vi "StatusReq20.vi"(1 "aDATA in":u8[](array[numeric])) -> ()   [LabVIEW 2017]
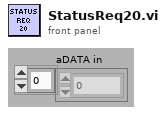
[diagram p1: front panel]
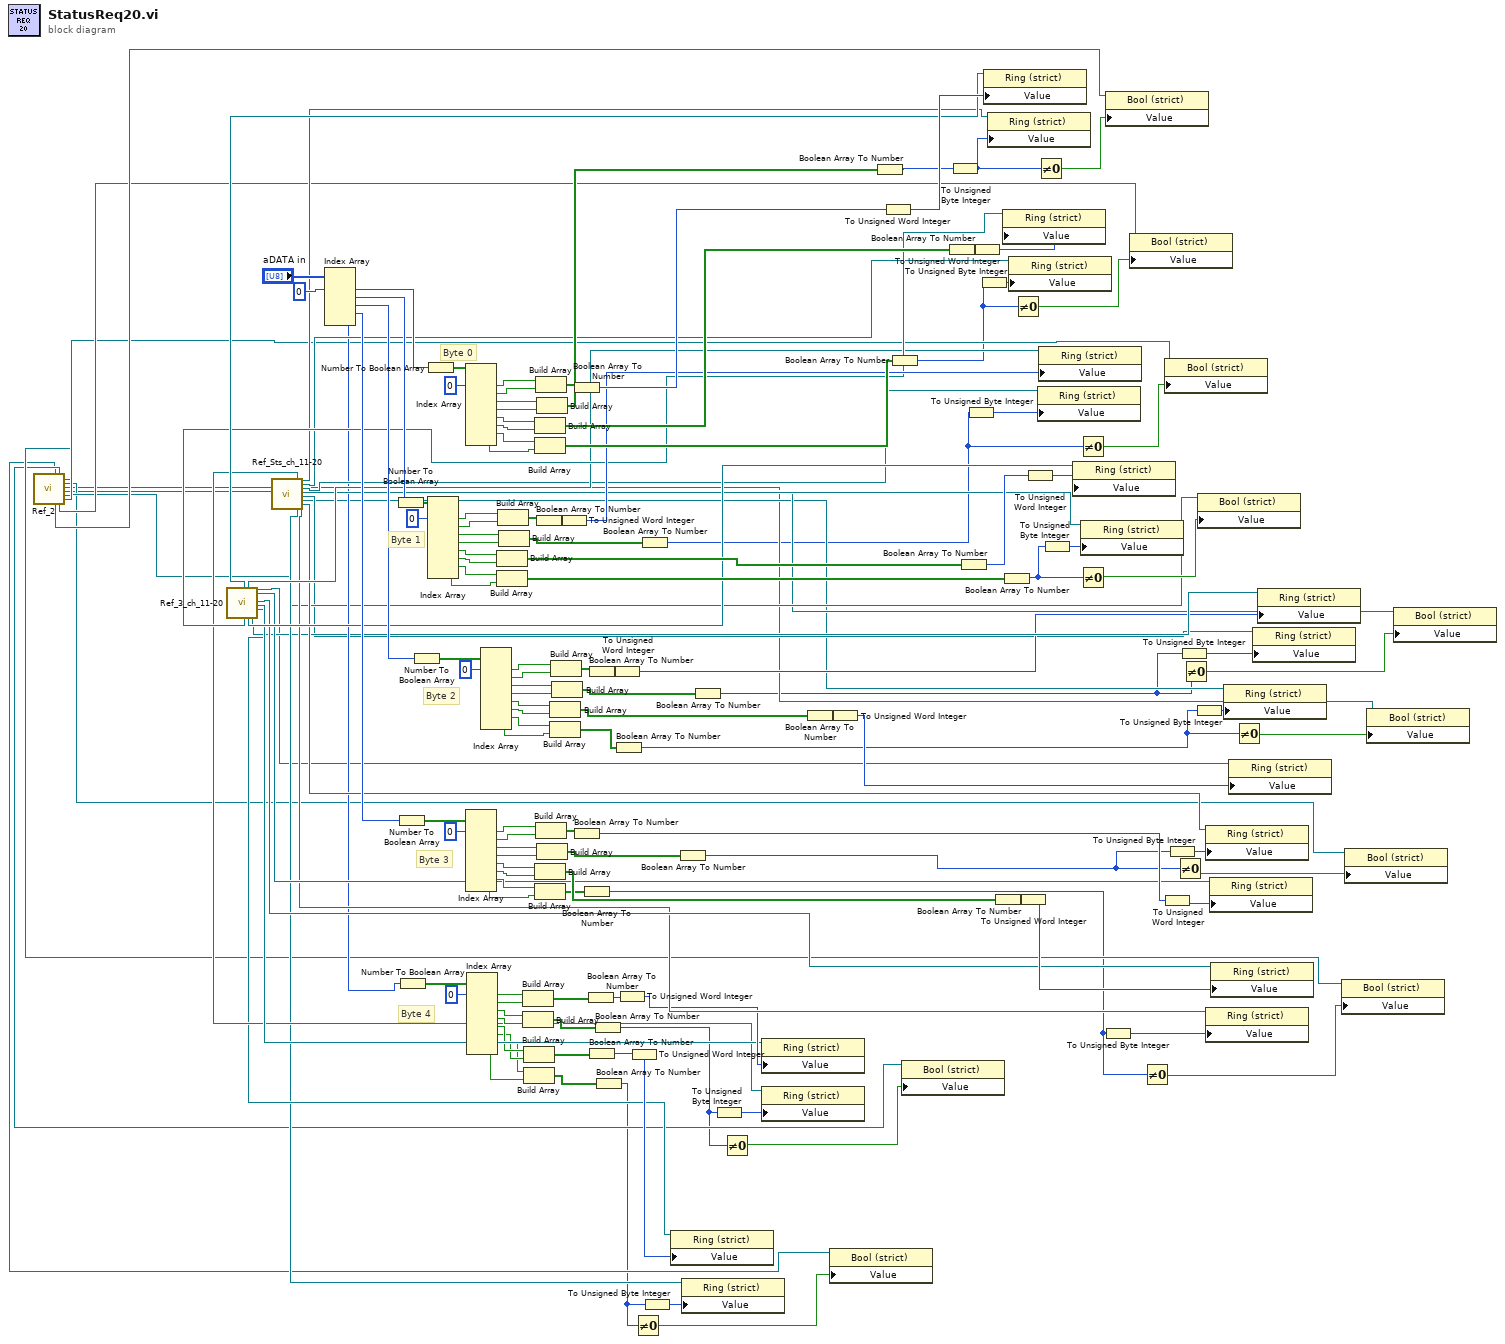
[diagram p0: block diagram]
diagram:
  # "Byte 4"
  # "Byte 3"
  # "Byte 2"
  # "Byte 1"
  # "Byte 0"
  n1 = call "Ref_2.vi"() -> ("Control  Ch 10 out"=w32:refnum<vi>, "Control  Ch 1 out"=w39:refnum<vi>, "Control  Ch 9 out"=w33:refnum<vi>, "Control  Ch 2 out"=w38:refnum<vi>, "Control  Ch 8 out"=w34:refnum<vi>, "Control  Ch 7 out"=w35:refnum<vi>, "Control  Ch 6 out"=w22:refnum<vi>, "Control  Ch 5 out"=w27:refnum<vi>, "Control  Ch 4 out"=w36:refnum<vi>, "Control  Ch 3 out"=w37:refnum<vi>)  [unwired: 17 in, 1 out]
  n2 = call "Ref_3_ch_11-20.vi"() -> ("Trip  Ch 11 out"=w81:refnum<vi>, "Trip  Ch 12 out"=w80:refnum<vi>, "Trip  Ch 13 out"=w79:refnum<vi>, "Trip  Ch 14 out"=w78:refnum<vi>, "Trip  Ch 15 out"=w31:refnum<vi>, "Trip  Ch 16 out"=w23:refnum<vi>, "Trip  Ch 17 out"=w77:refnum<vi>, "Trip  Ch 18 out"=w76:refnum<vi>, "Trip  Ch 19 out"=w58:refnum<vi>, "Trip  Ch 20 out"=w48:refnum<vi>)  [unwired: 18 in]
  n3 = call "Ref_Sts_ch_11-20.vi"() -> ("Status Ch 19 out"=w57:refnum<vi>, "Status Ch 20 out"=w47:refnum<vi>, "Status Ch 11 out"=w75:refnum<vi>, "Status Ch 12 out"=w74:refnum<vi>, "Status Ch 13 out"=w73:refnum<vi>, "Status Ch 14 out"=w72:refnum<vi>, "Status Ch 15 out"=w28:refnum<vi>, "Status Ch 16 out"=w24:refnum<vi>, "Status Ch 17 out"=w71:refnum<vi>, "Status Ch 18 out"=w70:refnum<vi>)  [unwired: 18 in]
  n4 = Index Array(array="aDATA in", index #1=0 ("index")) -> (element #1=w155:u8, element #2=w117:u8, element #3=w116:u8, element #4=w115:u8, element #5=w67:u8)  [unwired: 4 in]
  n5 = Number To Boolean Array(number=w117) -> (Boolean array=w135:bool[])
  n6 = Number To Boolean Array(number=w115) -> (Boolean array=w118:bool[])
  n7 = Number To Boolean Array(number=w67) -> (Boolean array=w69:bool[])
  n8 = Number To Boolean Array(number=w116) -> (Boolean array=w134:bool[])
  n9 = Number To Boolean Array(number=w155) -> (Boolean array=w154:bool[])
  n10 = Index Array(array=w135, index #1=0 ("index")) -> (element #1=w106:bool, element #2=w105:bool, element #3=w104:bool, element #4=w103:bool, element #5=w102:bool, element #6=w101:bool, element #7=w100:bool, element #8=w99:bool)  [unwired: 7 in]
  n11 = Index Array(array=w154, index #1=0 ("index")) -> (element #1=w114:bool, element #2=w113:bool, element #3=w112:bool, element #4=w111:bool, element #5=w110:bool, element #6=w109:bool, element #7=w108:bool, element #8=w107:bool)  [unwired: 7 in]
  n12 = Index Array(array=w118, index #1=0 ("index")) -> (element #1=w90:bool, element #2=w89:bool, element #3=w88:bool, element #4=w87:bool, element #5=w86:bool, element #6=w85:bool, element #7=w84:bool, element #8=w83:bool)  [unwired: 7 in]
  n13 = Index Array(array=w69, index #1=0 ("index")) -> (element #1=w65:bool, element #2=w66:bool, element #3=w64:bool, element #4=w63:bool, element #5=w52:bool, element #6=w51:bool, element #7=w50:bool, element #8=w49:bool)  [unwired: 7 in]
  n14 = Index Array(array=w134, index #1=0 ("index")) -> (element #1=w98:bool, element #2=w97:bool, element #3=w96:bool, element #4=w95:bool, element #5=w94:bool, element #6=w93:bool, element #7=w92:bool, element #8=w91:bool)  [unwired: 7 in]
  n15 = Build Array(w102, w101) -> (w143:bool[])
  n16 = Build Array(w100, w99) -> (w142:bool[])
  n17 = Build Array(w106, w105) -> (w137:bool[])
  n18 = Build Array(w104, w103) -> (w144:bool[])
  n19 = Build Array(w65, w66) -> (w61:bool[])
  n20 = Build Array(w64, w63) -> (w60:bool[])
  n21 = Build Array(w52, w51) -> (w54:bool[])
  n22 = Build Array(w50, w49) -> (w55:bool[])
  n23 = Boolean Array To Number(Boolean array=w137) -> (number=w138:u32)
  n24 = Build Array(w110, w109) -> (w146:bool[])
  n25 = Build Array(w108, w107) -> (w147:bool[])
  n26 = Build Array(w86, w85) -> (w125:bool[])
  n27 = Build Array(w84, w83) -> (w82:bool[])
  n28 = Build Array(w114, w113) -> (w152:bool[])
  n29 = Build Array(w90, w89) -> (w120:bool[])
  n30 = Build Array(w112, w111) -> (w145:bool[])
  n31 = Build Array(w88, w87) -> (w126:bool[])
  n32 = Build Array(w94, w93) -> (w128:bool[])
  n33 = Build Array(w92, w91) -> (w129:bool[])
  n34 = Build Array(w98, w97) -> (w132:bool[])
  n35 = Build Array(w96, w95) -> (w127:bool[])
  n36 = To Unsigned Word Integer(number=w138) -> (unsigned 16bit integer=w139:u16)
  n37 = Boolean Array To Number(Boolean array=w152) -> (number=w151:u32)
  n38 = Boolean Array To Number(Boolean array=w120) -> (number=w121:u32)
  n39 = Boolean Array To Number(Boolean array=w82) -> (number=w6:u32)
  n40 = Boolean Array To Number(Boolean array=w61) -> (number=w62:u32)
  n41 = Boolean Array To Number(Boolean array=w132) -> (number=w131:u32)
  n42 = Boolean Array To Number(Boolean array=w54) -> (number=w53:u32)
  n43 = Boolean Array To Number(Boolean array=w60) -> (number=w4:u32)
  n44 = Boolean Array To Number(Boolean array=w55) -> (number=w2:u32)
  n45 = To Unsigned Word Integer(number=w131) -> (unsigned 16bit integer=w30:u16)
  n46 = Boolean Array To Number(Boolean array=w129) -> (number=w10:u32)
  n47 = To Unsigned Word Integer(number=w62) -> (unsigned 16bit integer=w59:u16)
  n48 = To Unsigned Word Integer(number=w53) -> (unsigned 16bit integer=w56:u16)
  n49 = Not Equal To 0?(x=w2) -> (x != 0?=w46:bool)
  n50 = Boolean Array To Number(Boolean array=w144) -> (number=w18:u32)
  n51 = To Unsigned Byte Integer(number=w2) -> (unsigned 8bit integer=w1:u8)
  n52 = property class="Ring (strict)"(reference=w48, "Value"=w56) -> ()  [unwired: 1 in, 2 out]
  n53 = Boolean Array To Number(Boolean array=w126) -> (number=w8:u32)
  n54 = property class="Ring (strict)"(reference=w47, "Value"=w1) -> ()  [unwired: 1 in, 2 out]
  n55 = Boolean Array To Number(Boolean array=w127) -> (number=w12:u32)
  n56 = To Unsigned Byte Integer(number=w4) -> (unsigned 8bit integer=w3:u8)
  n57 = Not Equal To 0?(x=w4) -> (x != 0?=w45:bool)
  n58 = property class="Ring (strict)"(reference=w58, "Value"=w59) -> ()  [unwired: 1 in, 2 out]
  n59 = property class="Ring (strict)"(reference=w57, "Value"=w3) -> ()  [unwired: 1 in, 2 out]
  n60 = Boolean Array To Number(Boolean array=w128) -> (number=w130:u32)
  n61 = To Unsigned Word Integer(number=w130) -> (unsigned 16bit integer=w26:u16)
  n62 = property class="Bool (strict)"(reference=w32, "Value"=w46) -> ()  [unwired: 1 in, 2 out]
  n63 = Boolean Array To Number(Boolean array=w145) -> (number=w21:u32)
  n64 = To Unsigned Word Integer(number=w151) -> (unsigned 16bit integer=w150:u16)
  n65 = Boolean Array To Number(Boolean array=w147) -> (number=w14:u32)
  n66 = property class="Bool (strict)"(reference=w33, "Value"=w45) -> ()  [unwired: 1 in, 2 out]
  n67 = Boolean Array To Number(Boolean array=w146) -> (number=w149:u32)
  n68 = To Unsigned Byte Integer(number=w21) -> (unsigned 8bit integer=w20:u8)
  n69 = Boolean Array To Number(Boolean array=w143) -> (number=w140:u32)
  n70 = To Unsigned Byte Integer(number=w18) -> (unsigned 8bit integer=w17:u8)
  n71 = To Unsigned Word Integer(number=w149) -> (unsigned 16bit integer=w148:u16)
  n72 = To Unsigned Byte Integer(number=w14) -> (unsigned 8bit integer=w13:u8)
  n73 = property class="Ring (strict)"(reference=w81, "Value"=w150) -> ()  [unwired: 1 in, 2 out]
  n74 = property class="Ring (strict)"(reference=w75, "Value"=w20) -> ()  [unwired: 1 in, 2 out]
  n75 = Boolean Array To Number(Boolean array=w125) -> (number=w123:u32)
  n76 = Boolean Array To Number(Boolean array=w142) -> (number=w16:u32)
  n77 = property class="Ring (strict)"(reference=w80, "Value"=w148) -> ()  [unwired: 1 in, 2 out]
  n78 = property class="Ring (strict)"(reference=w74, "Value"=w13) -> ()  [unwired: 1 in, 2 out]
  n79 = Not Equal To 0?(x=w14) -> (x != 0?=w40:bool)
  n80 = To Unsigned Word Integer(number=w123) -> (unsigned 16bit integer=w124:u16)
  n81 = To Unsigned Word Integer(number=w140) -> (unsigned 16bit integer=w141:u16)
  n82 = Not Equal To 0?(x=w20) -> (x != 0?=w19:bool)
  n83 = property class="Ring (strict)"(reference=w73, "Value"=w17) -> ()  [unwired: 1 in, 2 out]
  n84 = property class="Ring (strict)"(reference=w79, "Value"=w139) -> ()  [unwired: 1 in, 2 out]
  n85 = To Unsigned Byte Integer(number=w16) -> (unsigned 8bit integer=w15:u8)
  n86 = property class="Ring (strict)"(reference=w78, "Value"=w141) -> ()  [unwired: 1 in, 2 out]
  n87 = Not Equal To 0?(x=w18) -> (x != 0?=w41:bool)
  n88 = Not Equal To 0?(x=w16) -> (x != 0?=w42:bool)
  n89 = property class="Ring (strict)"(reference=w72, "Value"=w15) -> ()  [unwired: 1 in, 2 out]
  n90 = To Unsigned Byte Integer(number=w6) -> (unsigned 8bit integer=w5:u8)
  n91 = property class="Bool (strict)"(reference=w39, "Value"=w19) -> ()  [unwired: 1 in, 2 out]
  n92 = property class="Bool (strict)"(reference=w38, "Value"=w40) -> ()  [unwired: 1 in, 2 out]
  n93 = Not Equal To 0?(x=w6) -> (x != 0?=w44:bool)
  n94 = To Unsigned Word Integer(number=w121) -> (unsigned 16bit integer=w122:u16)
  n95 = property class="Bool (strict)"(reference=w37, "Value"=w41) -> ()  [unwired: 1 in, 2 out]
  n96 = To Unsigned Byte Integer(number=w8) -> (unsigned 8bit integer=w7:u8)
  n97 = Not Equal To 0?(x=w8) -> (x != 0?=w43:bool)
  n98 = To Unsigned Byte Integer(number=w12) -> (unsigned 8bit integer=w11:u8)
  n99 = Not Equal To 0?(x=w12) -> (x != 0?=w29:bool)
  n100 = To Unsigned Byte Integer(number=w10) -> (unsigned 8bit integer=w9:u8)
  n101 = property class="Bool (strict)"(reference=w36, "Value"=w42) -> ()  [unwired: 1 in, 2 out]
  n102 = property class="Ring (strict)"(reference=w71, "Value"=w7) -> ()  [unwired: 1 in, 2 out]
  n103 = property class="Ring (strict)"(reference=w70, "Value"=w5) -> ()  [unwired: 1 in, 2 out]
  n104 = property class="Ring (strict)"(reference=w77, "Value"=w122) -> ()  [unwired: 1 in, 2 out]
  n105 = property class="Ring (strict)"(reference=w76, "Value"=w124) -> ()  [unwired: 1 in, 2 out]
  n106 = property class="Ring (strict)"(reference=w24, "Value"=w9) -> ()  [unwired: 1 in, 2 out]
  n107 = property class="Ring (strict)"(reference=w23, "Value"=w26) -> ()  [unwired: 1 in, 2 out]
  n108 = Not Equal To 0?(x=w10) -> (x != 0?=w25:bool)
  n109 = property class="Ring (strict)"(reference=w28, "Value"=w11) -> ()  [unwired: 1 in, 2 out]
  n110 = property class="Ring (strict)"(reference=w31, "Value"=w30) -> ()  [unwired: 1 in, 2 out]
  n111 = property class="Bool (strict)"(reference=w34, "Value"=w44) -> ()  [unwired: 1 in, 2 out]
  n112 = property class="Bool (strict)"(reference=w35, "Value"=w43) -> ()  [unwired: 1 in, 2 out]
  n113 = property class="Bool (strict)"(reference=w22, "Value"=w25) -> ()  [unwired: 1 in, 2 out]
  n114 = property class="Bool (strict)"(reference=w27, "Value"=w29) -> ()  [unwired: 1 in, 2 out]
